vi "Initialize Routing Channel Page (Route Configuration).vi"(8 "error in (no error)":errorcluster, 10 "Routing Channel Page Controls":T1, 11 "Routing Channel Ref in":T2 format="%.0x") -> (0 "error out":errorcluster, 3 "Routing Channel Ref out":T2 format="%.0x")   [LabVIEW 2017, in "Routing and Faulting System Explorer.lvlib"]
uses:
  Routing and Faulting System Explorer.lvlib
  <vilib>/NI Veristand/Custom Device API/Custom Device Item Ref.ctl
  Routing Channel Page Controls.ctl
  Scripting/Switch Scripting.lvlib
  <vilib>/NI VeriStand/Custom Device API/Custom Device API.lvlib
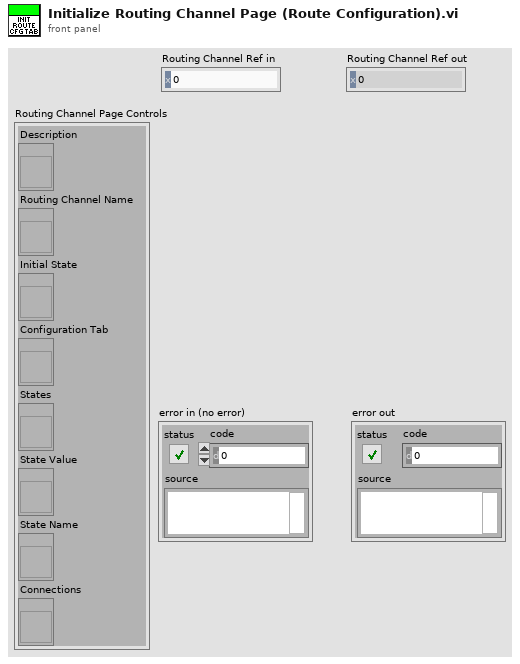
[diagram p1: front panel]
types:
  T1 = typedef "Routing and Faulting System Explorer.lvlib/Routing Channel Page Controls.ctl" = cluster{"Description":refnum<vi>, "Routing Channel Name":refnum<vi>, "Initial State":refnum<vi>, "Configuration Tab":refnum<vi>, "States":refnum<vi>, "State Value":refnum<vi>, "State Name":refnum<vi>, "Connections":refnum<vi>}
  T2 = typedef "Custom Device API.lvlib/Custom Device Item Ref.ctl" = u64
  T3 = enum8{"Enabled", "Disabled", "Disabled and Grayed Out"}
  T4 = typedef "Routing and Faulting Shared.lvlib/Routing State.ctl" = cluster{"Name":string, "Description":string, "Value":i32, "Connection List":T5[]}
  T5 = typedef "Routing and Faulting Shared.lvlib/Connection.ctl" = cluster{"Resource":string, "Source":string, "Destination":string}
  T6 = typedef "Routing and Faulting System Explorer.lvlib/Connection Row.ctl" = cluster{"Source":string, "Destination":string}
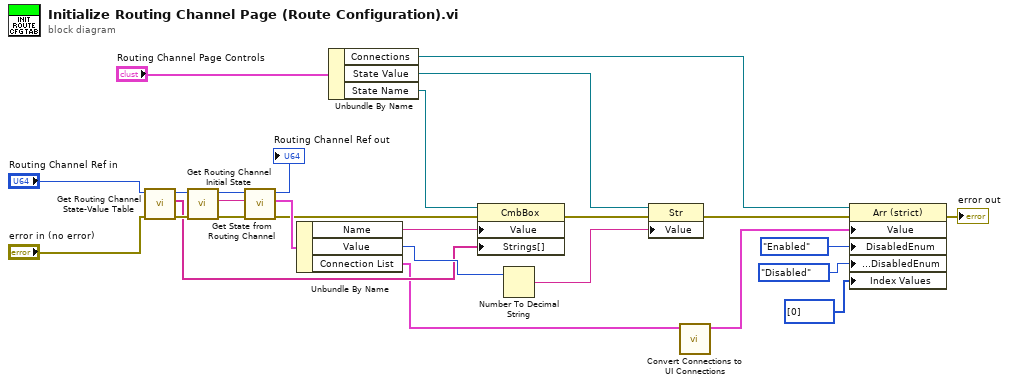
[diagram p0: block diagram]
diagram:
  n1 = call "Get Routing Channel State-Value Table.vi"("error in (no error)"="error in (no error)", "Channel Ref in"="Routing Channel Ref in") -> ("error out"=w25:errorcluster, "State Names"=w7:string[], "Channel Ref out"=w26:T2)  [unwired: 6 in, 1 out]
  n2 = call "Get Routing Channel Initial State.vi"("error in (no error)"=w25, "Channel Ref in"=w26) -> ("error out"=w3:errorcluster, "Initial State"=w22:string, "Channel Ref out"=w4:T2)  [unwired: 7 in]
  n3 = call "Get State from Routing Channel.vi"("error in (no error)"=w3, "State"=w22, "Channel Ref in"=w4) -> ("error out"=w20:errorcluster, "State and Connections"=w21:T4, "Channel Ref out"=→"Routing Channel Ref out":T2)  [unwired: 6 in]
  n4 = Unbundle By Name(w21) -> ("Name"=w19:string, "Value"=w17:i32, "Connection List"=w2:T5[])
  n5 = Unbundle By Name("Routing Channel Page Controls") -> ("Connections"=w11:refnum<vi>, "State Value"=w12:refnum<vi>, "State Name"=w13:refnum<vi>)
  n6 = property class="CmbBox"(reference=w13, error in=w20, "Value"=w19, "Strings[]"=w7) -> (error out=w18:errorcluster)  [unwired: 1 out]
  n7 = Number To Decimal String(number=w17) -> (decimal integer string=w16:string)  [unwired: 1 in]
  n8 = property class="Str"(reference=w12, error in=w18, "Value"=w16) -> (error out=w15:errorcluster)  [unwired: 1 out]
  n9 = call "Convert Connections to UI Connections.vi"("Connection List"=w2) -> ("UI Connections List"=w1:T6[])  [unwired: 10 in]
  n10 = property class="Arr (strict)"(reference=w11, error in=w15, "Value"=w1, "DisabledEnum"=T3."Enabled" ("Disabled"), "Array Element.DisabledEnum"=T3."Disabled" ("Array Element.Disabled"), "Index Values"=u32[] [0]) -> (error out=→"error out":errorcluster)  [unwired: 1 out]
